vi "BoxBegin.vi"(8 "error in (no error)":errorcluster) -> (0 "error out":errorcluster)   [LabVIEW 2023]
uses:
  <vilib>/Rock Robotics/SystemInterfaces/DIO/FPGA_DIOChannel.ctl
  <vilib>/Rock Robotics/WPI/ThirdParty/REV Robotics/REVLib/Typedef/Spark MAX Sensor Type.ctl
  <vilib>/Rock Robotics/WPI/ThirdParty/REV Robotics/REVLib/Typedef/Spark MAX Idle Mode.ctl
  <vilib>/Rock Robotics/WPI/ThirdParty/REV Robotics/REVLib/Typedef/Spark MAX Motor Type.ctl
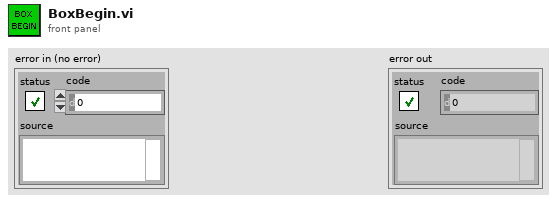
[diagram p1: front panel]
types:
  T1 = typedef "FPGA_DIOChannel.ctl" = enum8{"DIO 0", "DIO 1", "DIO 2", "DIO 3", "DIO 4", "DIO 5", "DIO 6", "DIO 7", "DIO 8", "DIO 9", "DIO MXP 0", "DIO MXP 1", "DIO MXP 2", "DIO MXP 3", "DIO MXP 4", "DIO MXP 5", "DIO MXP 6", "DIO MXP 7", "DIO MXP 8", "DIO MXP 9", "DIO MXP 10", "DIO MXP 11", "DIO MXP 12", "DIO MXP 13", "DIO MXP 14", "DIO MXP 15", "SPI Port CS1", "SPI Port CS2", "SPI Port CS3", "SPI Port MISO", "SPI Port MOSI", "Invalid"}
  T2 = typedef "Spark MAX Sensor Type.ctl" = enum16{"No Sensor", "Hall Sensor", "Encoder", "-Not Available-", "Analog", "Alternate Encoder", "Duty Cycle"}
  T3 = typedef "Spark MAX Idle Mode.ctl" = enum16{"Coast", "Brake"}
  T4 = typedef "Spark MAX Motor Type.ctl" = enum16{"Brushed", "Brushless"}
  T5 = typedef "WPI_DigitalInputDevRef.ctl" = cluster{"DevStatus":errorcluster, "DIO Channel":T1}
  T6 = typedef "WPI_MotorControlDeviceRef.ctl" = cluster{"DeviceStatus":errorcluster, "Type":T7, "PWM":cluster{"PWM Channel":T8, "DeadBand":T9}, "CAN":cluster{"Device Number":u8, "SetOutput VI Ref":variant, "GetOutput VI Ref":variant, "Enable VI Ref":variant, "Disable VI Ref":variant, "Data":variant}, "Invert":bool, "DIO PWM":cluster{"PWM \"Enable\" Channel":T8, "DIOChannel":T1, "PWM Rate":dbl}}
  T7 = typedef "WPI_MotorControlType.ctl" = enum16{"PWM", "CAN", "DIO PWM"}
  T8 = typedef "FPGA_DIOPWMChannel.ctl" = enum8{"PWM 0", "PWM 1", "PWM 2", "PWM 3", "PWM 4", "PWM 5", "PWM 6", "PWM 7", "PWM 8", "PWM 9", "PWM MXP 0", "PWM MXP 1", "PWM MXP 2", "PWM MXP 3", "PWM MXP 4", "PWM MXP 5", "PWM MXP 6", "PWM MXP 7", "PWM MXP 8", "PWM MXP 9", "Invalid"}
  T9 = typedef "WPI_PWMDeadband.ctl" = cluster{"Name":string, "maxPositivePwm":i32, "minPositivePwm":i32, "centerPwm":i32, "maxNegativePwm":i32, "minNegativePwm":i32, "angularRange":u16}
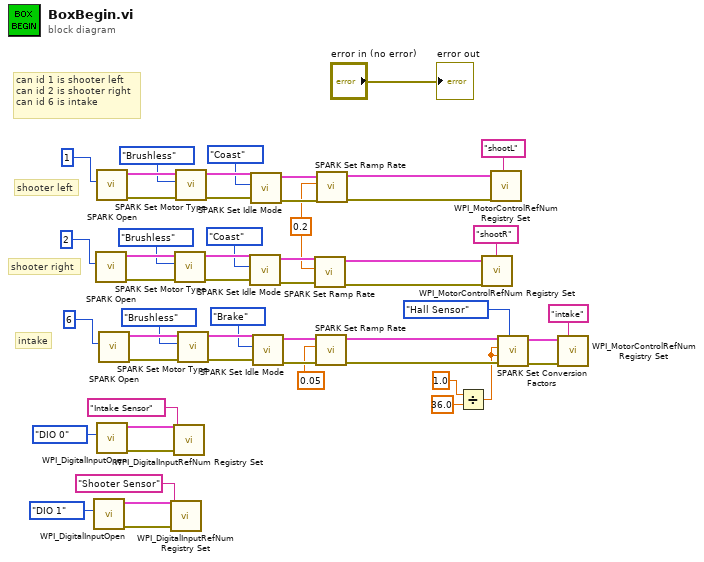
[diagram p0: block diagram]
diagram:
  w23 = 0.2
  # "intake"
  # "shooter right"
  # "shooter left"
  # "can id 1 is shooter left\ncan id 2 is shooter right\ncan id 6 is intake"
  n1 = call <vilib>:"WPI_DigitalInputOpen.vi"("DIO Channel"=FPGA_DIOChannel."DIO 1") -> ("error out"=w4:errorcluster, "DigitalInputDevRef"=w3:T5)  [unwired: 9 in]
  n2 = call <vilib>:"SPARK Open.vi"("Device Number"=2) -> ("error out"=w41:errorcluster, "MotorControlDeviceRef"=w43:T6)  [unwired: 9 in]
  n3 = call <vilib>:"SPARK Open.vi"("Device Number"=1) -> ("error out"=w49:errorcluster, "MotorControlDeviceRef"=w51:T6)  [unwired: 9 in]
  n4 = call <vilib>:"WPI_DigitalInputOpen.vi"("DIO Channel"=FPGA_DIOChannel."DIO 0") -> ("error out"=w8:errorcluster, "DigitalInputDevRef"=w7:T5)  [unwired: 9 in]
  n5 = call <vilib>:"SPARK Open.vi"("Device Number"=6) -> ("error out"=w33:errorcluster, "MotorControlDeviceRef"=w35:T6)  [unwired: 9 in]
  n6 = call <vilib>:"WPI_DigitalInputRefNum Registry Set.vi"("error in (no error)"=w4, "refnum name"="Shooter Sensor", "DigitalInputDevRef"=w3) -> ()  [unwired: 7 in, 2 out]
  n7 = call <vilib>:"WPI_DigitalInputRefNum Registry Set.vi"("error in (no error)"=w8, "refnum name"="Intake Sensor", "DigitalInputDevRef"=w7) -> ()  [unwired: 7 in, 2 out]
  n8 = call <vilib>:"SPARK Set Motor Type.vi"("error in (no error)"=w41, "Motor Type"=Spark_MAX_Motor_Type."Brushless", "MotorControlDevRef"=w43) -> ("error out"=w40:errorcluster, "MotorControlDeviceRef"=w42:T6)  [unwired: 7 in]
  n9 = call <vilib>:"SPARK Set Motor Type.vi"("error in (no error)"=w49, "Motor Type"=Spark_MAX_Motor_Type."Brushless", "MotorControlDevRef"=w51) -> ("error out"=w48:errorcluster, "MotorControlDeviceRef"=w50:T6)  [unwired: 7 in]
  n10 = call <vilib>:"SPARK Set Motor Type.vi"("error in (no error)"=w33, "Motor Type"=Spark_MAX_Motor_Type."Brushless", "MotorControlDevRef"=w35) -> ("error out"=w32:errorcluster, "MotorControlDeviceRef"=w34:T6)  [unwired: 7 in]
  n11 = call <vilib>:"SPARK Set Idle Mode.vi"("error in (no error)"=w40, "Idle Mode"=Spark_MAX_Idle_Mode."Coast", "MotorControlDeviceRef in"=w42) -> ("error out"=w28:errorcluster, "MotorControlDeviceRef out"=w29:T6)  [unwired: 7 in]
  n12 = call <vilib>:"SPARK Set Idle Mode.vi"("error in (no error)"=w48, "Idle Mode"=Spark_MAX_Idle_Mode."Coast", "MotorControlDeviceRef in"=w50) -> ("error out"=w27:errorcluster, "MotorControlDeviceRef out"=w26:T6)  [unwired: 7 in]
  n13 = call <vilib>:"SPARK Set Idle Mode.vi"("error in (no error)"=w32, "Idle Mode"=Spark_MAX_Idle_Mode."Brake", "MotorControlDeviceRef in"=w34) -> ("error out"=w24:errorcluster, "MotorControlDeviceRef out"=w25:T6)  [unwired: 7 in]
  n14 = call <vilib>:"SPARK Set Ramp Rate.vi"("error in (no error)"=w28, "Seconds from neutral to full (0)"=w23, "MotorControlDeviceRef in"=w29) -> ("error out"=w15:errorcluster, "MotorControlDeviceRef"=w14:T6)  [unwired: 7 in]
  n15 = call <vilib>:"SPARK Set Ramp Rate.vi"("error in (no error)"=w24, "Seconds from neutral to full (0)"=0.05, "MotorControlDeviceRef in"=w25) -> ("error out"=w17:errorcluster, "MotorControlDeviceRef"=w16:T6)  [unwired: 7 in]
  n16 = call <vilib>:"SPARK Set Ramp Rate.vi"("error in (no error)"=w27, "Seconds from neutral to full (0)"=w23, "MotorControlDeviceRef in"=w26) -> ("error out"=w18:errorcluster, "MotorControlDeviceRef"=w19:T6)  [unwired: 7 in]
  n17 = Divide(x=1.0, y=36.0) -> (x/y=w10:dbl)
  n18 = call <vilib>:"WPI_MotorControlRefNum Registry Set.vi"("error in (no error)"=w15, "refnum name"="shootR", "MotorControlDevRef"=w14) -> ()  [unwired: 7 in, 2 out]
  n19 = call <vilib>:"WPI_MotorControlRefNum Registry Set.vi"("error in (no error)"=w18, "refnum name"="shootL", "MotorControlDevRef"=w19) -> ()  [unwired: 7 in, 2 out]
  n20 = call <vilib>:"SPARK Set Conversion Factors.vi"("Sensor Type (Hall Sensor)"=Spark_MAX_Sensor_Type."Hall Sensor", "error in (no error)"=w17, "Velocity Factor (1)"=w10, "Position Factor (1)"=w10, "MotorControlDeviceRef in"=w16) -> ("error out"=w20:errorcluster, "MotorControlDeviceRef out"=w21:T6)  [unwired: 5 in]
  n21 = call <vilib>:"WPI_MotorControlRefNum Registry Set.vi"("error in (no error)"=w20, "refnum name"="intake", "MotorControlDevRef"=w21) -> ()  [unwired: 7 in, 2 out]
  "error out" <- "error in (no error)"
